vi "Network Application Folder.vi"(4 "Force App? (f)":bool, 5 "error in (no error)":errorcluster, 6 "App reference (NULL)":refnum<vi>) -> (0 "LabVIEW Application Network Path":path, 1 "error out":errorcluster, 2 "dup App reference":refnum<vi>)   [LabVIEW 2011]
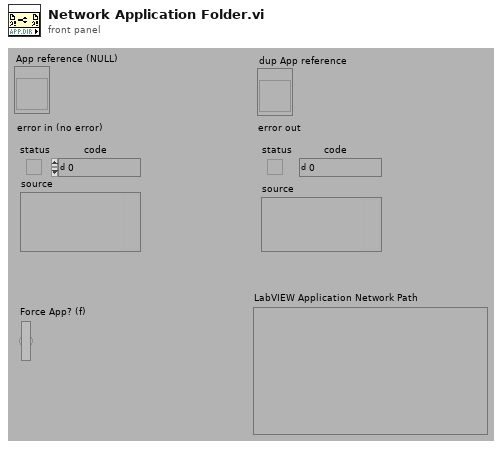
[diagram p1: front panel]
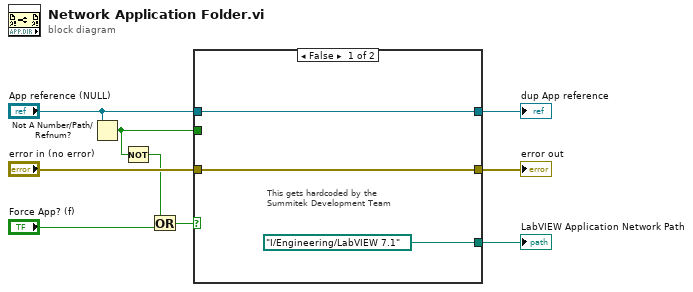
[diagram p0: block diagram]
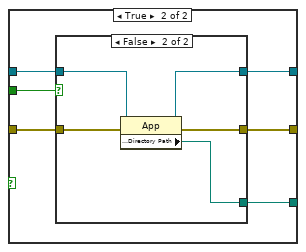
[diagram p2: hidden frame]
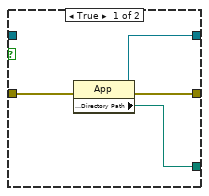
[diagram p3: hidden frame]
diagram:
  n1 = Not A Number/Path/Refnum?(number/path/refnum="App reference (NULL)") -> (NaN/Path/Refnum?=w1:bool)
  n2 = Not(x=w1) -> (.not. x?=w4:bool)
  n3 = Or(x=w4, y="Force App? (f)") -> (x .or. y?=w2:bool)
  n4 = case shown="False" w2 {
    tunnel: "App reference (NULL)" -> [w12 w14]
    tunnel: "error in (no error)" -> [w11 w18]
    tunnel: [w11 w17] -> w8
    tunnel: [w12 w16] -> w7
    tunnel: [path "I:/Engineering/LabVIEW 7.1" ("App.Dir") w15] -> w6
    tunnel: w1 -> [_ w13]
    frame False {
      # "This gets hardcoded by the\nSummitek Development Team"
    }
    frame True {
      n5 = case shown="False" w13 {
        tunnel: w18 -> [w22 w27]
        tunnel: [w21 w26] -> w17
        tunnel: [w20 w25] -> w16
        tunnel: [w19 w24] -> w15
        tunnel: w14 -> [_ w23]
        frame True {
          n6 = property class="App"(error in=w22) -> (reference out=w20:refnum<vi>, error out=w21:errorcluster, "Application:Directory Path"=w19:path)  [unwired: 1 in]
        }
        frame False {
          n7 = property class="App"(reference=w23, error in=w27) -> (reference out=w25:refnum<vi>, error out=w26:errorcluster, "Application:Directory Path"=w24:path)
        }
      }
    }
  }
  "LabVIEW Application Network Path" <- w6
  "dup App reference" <- w7
  "error out" <- w8
